vi "Format Library Control VI Info Table.vi"(7 "Methods":T1, 8 "Error in":errorcluster caption="Error in (no error)", 9 "Msg Chain":string, 10 "VI Info Array":T2[](array[typedef]), 11 "VIDoc Printer - Confluence In":refnum<class "VIDoc Printer - Confluence.lvclass">) -> (0 "Error out":errorcluster, 2 "Table String":string, 3 "VIDoc Printer - Confluence Out":refnum<class "VIDoc Printer - Confluence.lvclass">)   [LabVIEW 2023, in "VIDoc Printer - Confluence.lvlib" / "VIDoc Printer - Confluence.lvclass"]
uses:
  VIDoc Printer - Confluence.lvclass
  Parsing/TypeDefs/Method Spec Cluster.ctl
  Parsing/TypeDefs/VI Type Extended Enum.ctl
  <vilib>/picture/picture.llb/imagedata.ctl
  Parsing/TypeDefs/Class Dispatch Type Enum.ctl
  Parsing/TypeDefs/Controls Info Cluster.ctl
  <vilib>/Utility/miscctls.llb/LVKeyTypeDef.ctl
  <vilib>/Utility/miscctls.llb/LVPointTypeDef.ctl
  Parsing/SubVIs/Structure Reporter/Tree Cluster.ctl
  Settings/Printer Settings/Detail Level Enum.ctl
  C:/projects/DMC/Tooling/Git-Action-Service/Source/Documentation Generation/Printers/Printer/VIDoc Printer.lvclass
  VIDoc Printer - Confluence.lvclass/VIDoc Printer - Confluence.ctl
  Printer/VIDoc Printer.lvclass/VIDoc Printer.ctl
  Printer/Accessors/Get Formatting Settings - Bookmark Options.vi
  Accessors/Get Temporary Image Directory+.vi
  Accessors/Get Control Method Column Ordering - Full.vi
  Accessors/Get Control Method Column Ordering - Minimal.vi
  Accessors/Get Control Method Column Ordering - Standard.vi
  Accessors/Get Sortable Tables.vi
  <vilib>/Utility/libraryn.llb/Create Directory Recursive.vi
  Printer/VIDoc Printer.lvclass
  Confluence Formatting/Confluence Formatting.lvlib
  UI Interaction/UI Interaction.lvclass
  C:/projects/DMC/Tooling/Git-Action-Service/Source/Documentation Generation/Printers/Confluence Printer/VIDoc Printer - Confluence.lvclass
  Parsing/VIDoc Parsing.lvlib
  Settings/Printer Settings/Printer Settings.lvclass
  Parsing/SubVIs/Structure Reporter/Structure Reporter.lvlib
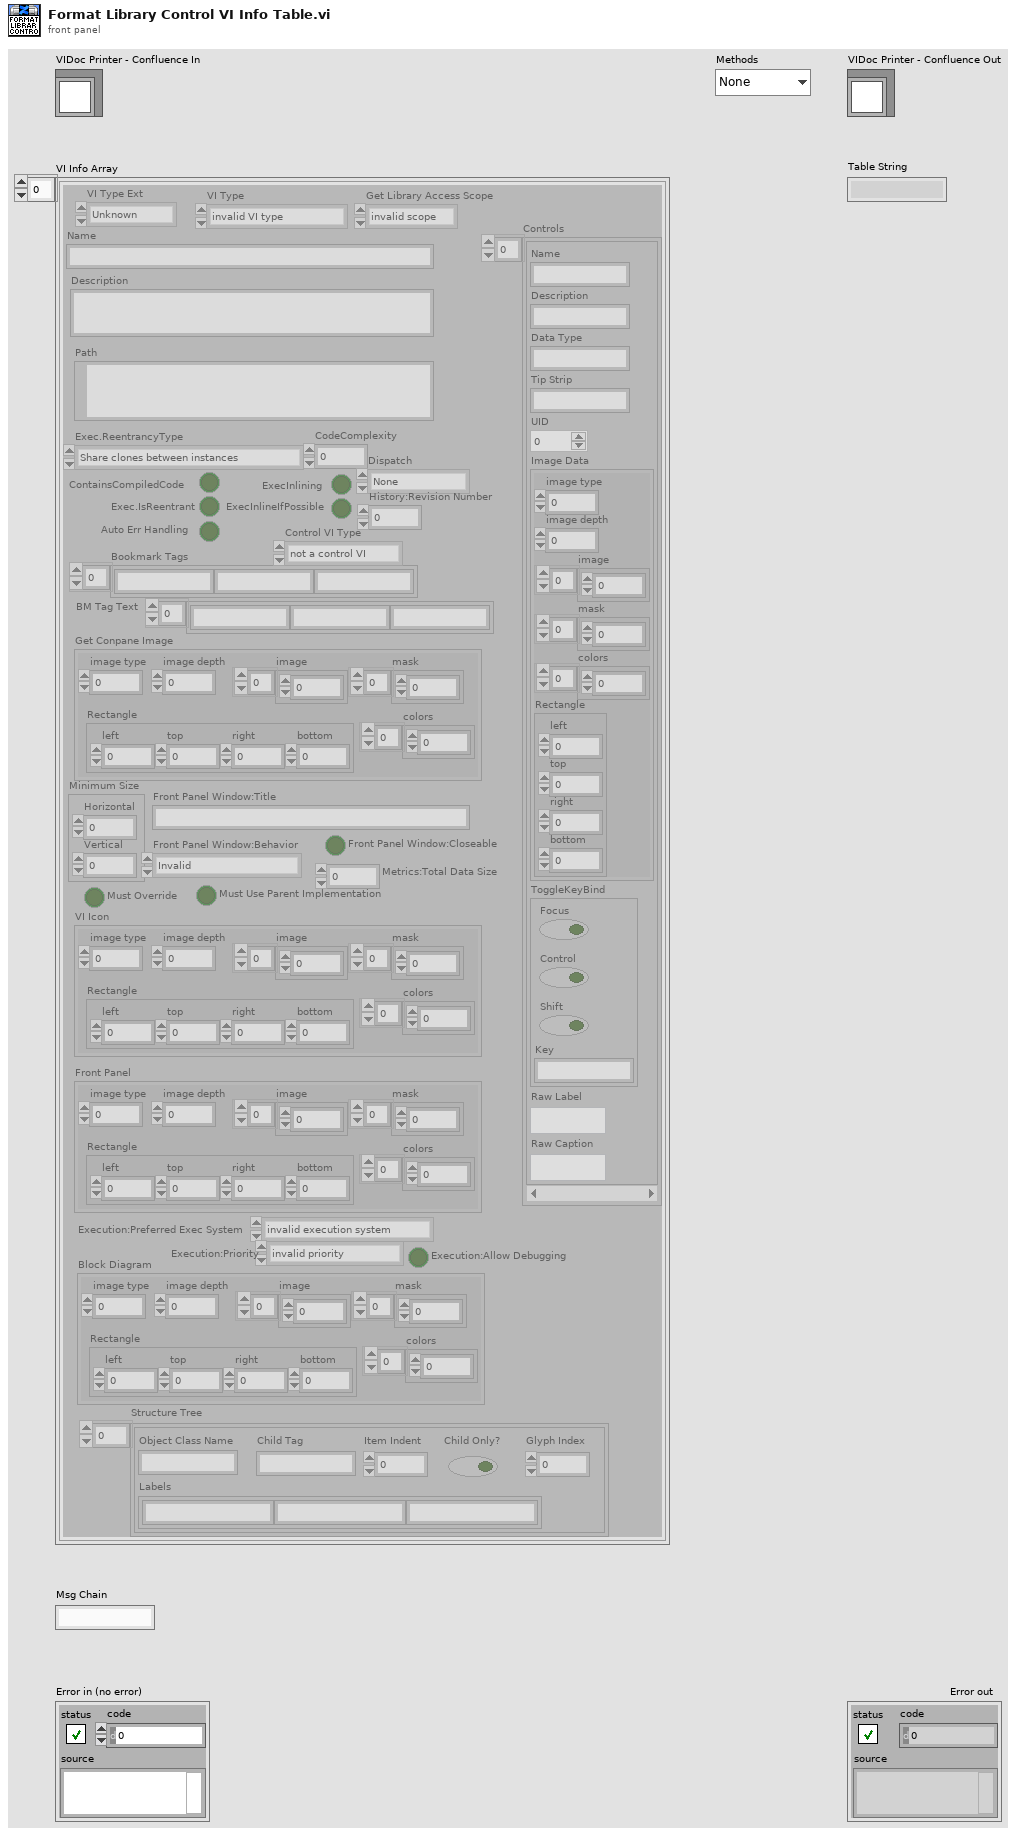
[diagram p1: front panel]
types:
  T1 = typedef "VIDoc Printer.lvlib/Printer Settings.lvclass/Detail Level Enum.ctl" = enum16{"None", "Minimal", "Standard", "Full"}
  T2 = typedef "VIDoc Parsing.lvlib/Method Spec Cluster.ctl" = cluster{"VI Type Ext":T3, "Name":string, "Path":path, "Get Conpane Image":T4, "Description":string, "Get Library Access Scope":enum32{"invalid scope", "public", "private", "protected", "community"}, "Dispatch":T5, "ContainsCompiledCode":bool, "Exec.IsReentrant":bool, "Exec.ReentrancyType":enum16{"Share clones between instances", "Preallocate clone for each instance"}, "ExecInlining":bool, "ExecInlineIfPossible":bool, "Auto Err Handling":bool, "CodeComplexity":sgl, "Bookmark Tags":string[], "Control VI Type":enum32{"not a control VI", "control", "typedef", "strict typedef"}, "Controls":T6[], "VI Type":enum32{"invalid VI type", "Standard VI", "Control VI", "Global VI", "Polymorphic VI", "Configuration VI", "SubSystem", "Facade VI", "Method VI", "Statechart Diagram VI"}, "Minimum Size":T8, "Front Panel Window:Title":string, "Front Panel Window:Behavior":enum32{"Invalid", "Default", "Floating", "Floating/Auto-Hide", "Modal"}, "Front Panel Window:Closeable":bool, "Must Override":bool, "Must Use Parent Implementation":bool, "VI Icon":T4, "Front Panel":T4, "History:Revision Number":u32, "Metrics:Total Data Size":u32, "Execution:Allow Debugging":bool, "Execution:Preferred Exec System":enum32{"invalid execution system", "user interface", "standard", "instrument i/o", "data acquisition", "other 1", "other 2", "same as caller"}, "Execution:Priority":enum32{"invalid priority", "background priority", "normal priority", "above normal priority", "high priority", "time critical priority", "subroutine"}, "BM Tag Text":string[], "Block Diagram":T4, "Structure Tree":T9[]}
  T3 = typedef "VIDoc Parsing.lvlib/VI Type Extended Enum.ctl" = enum16{"Unknown", "Class Method", "Class Accessor Get", "Class Accessor Set", "Class Control", "Library Method", "Library Control", "VI", "Control"}
  T4 = typedef "imagedata.ctl" = cluster{"image type":i32, "image depth":i32, "image":u8[], "mask":u8[], "colors":u32[], "Rectangle":cluster{"left":i16, "top":i16, "right":i16, "bottom":i16}}
  T5 = typedef "VIDoc Parsing.lvlib/Class Dispatch Type Enum.ctl" = enum16{"None", "Static", "Dynamic"}
  T6 = typedef "VIDoc Parsing.lvlib/Controls Info Cluster.ctl" = cluster{"Name":string, "Description":string, "Data Type":string, "Tip Strip":string, "UID":i32, "Image Data":T4, "ToggleKeyBind":T7, "Raw Label":string, "Raw Caption":string}
  T7 = typedef "LVKeyTypeDef.ctl" = cluster{"Focus":bool, "Control":bool, "Shift":bool, "Key":string}
  T8 = typedef "LVPointTypeDef.ctl" = cluster{"Horizontal":i16, "Vertical":i16}
  T9 = typedef "VIDoc Parsing.lvlib/Structure Reporter.lvlib/Tree Cluster.ctl" = cluster{"Object Class Name":string, "Labels":string[], "Child Tag":string, "Item Indent":i32, "Child Only?":bool, "Glyph Index":i32}
  T10 = enum32{"invalid scope", "public", "private", "protected", "community"}
  T11 = enum32{"not a control VI", "control", "typedef", "strict typedef"}
  T12 = typedef "VIDoc Printer.lvlib/Printer Settings.lvclass/Bookmark Options.ctl" = cluster{"Bookmarks as New Line in VI Descriptions":bool, "Unique Bookmark Tags Only":bool, "Include Tag and Text":bool}
  T13 = typedef "VIDoc Printer - Confluence.lvlib/VIDoc Settings - Confluence.lvclass/VI Info Column.ctl" = enum16{"Name", "Conpane", "BD", "FP", "VI Icon", "Description", "Reentrant", "Inline", "Auto Error", "Compiled", "Code Complexity", "Data Size", "Debug", "Priority", "Rev", "Minimum Size", "Title", "FP Behavior", "FP Closeable", "Author", "Commit Hash", "Last Change", "Branch", "Scope", "Type", "Dispatch", "Must Override", "Must Use Parent", "Structure Tree"}
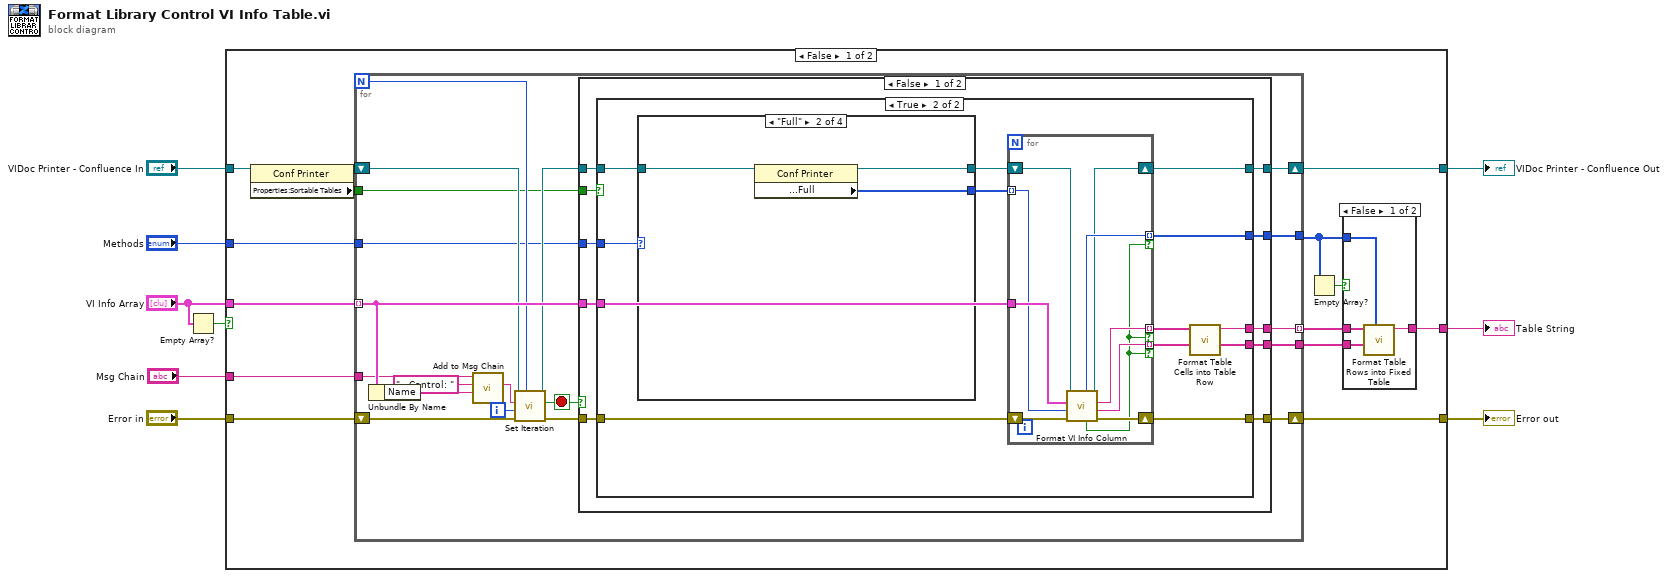
[diagram p0: block diagram]
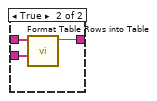
[diagram p2: hidden frame]
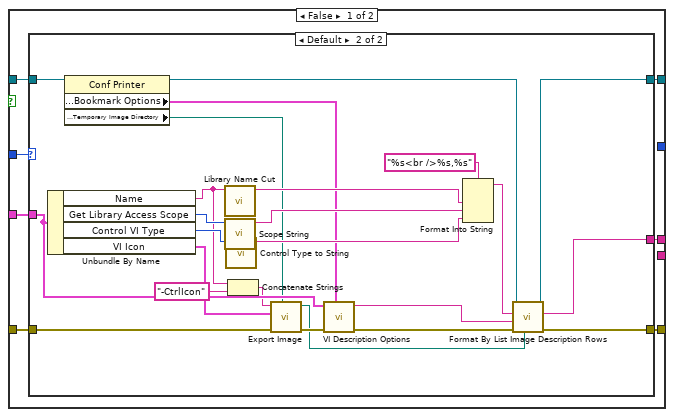
[diagram p3: hidden frame]
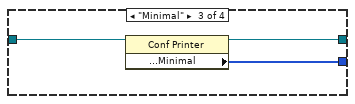
[diagram p6: hidden frame]
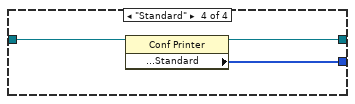
[diagram p7: hidden frame]
diagram:
  n1 = Empty Array?(array="VI Info Array") -> (empty?=w1:bool)
  n2 = case shown="False" w1 {
    tunnel: "Error in" -> [w23 w127]
    tunnel: [w22 w127] -> w8
    tunnel: [w21 _] -> w7
    tunnel: "VI Info Array" -> [w20 _]
    tunnel: "VIDoc Printer - Confluence In" -> [w19 w128]
    tunnel: [w18 w128] -> w5
    tunnel: "Msg Chain" -> [w17 _]
    tunnel: "Methods" -> [w16 _]
    frame False {
      n3 = property class="Conf Printer"(reference=w19) -> (reference out=w11:refnum<class "VIDoc Printer - Confluence.lvclass">, "Properties:Sortable Tables"=w10:bool)  [unwired: 1 in, 1 out]
      n4 = for {
        N -> [w40]
        tunnel: w20 -> [w43] mode=indexing
        shift-right: [w49] -> w18
        shift-left: w11 -> [w38]
        shift-right: [w48] -> w22
        shift-left: w23 -> [w45]
        tunnel: w17 -> [w41]
        tunnel: w16 -> [w35]
        tunnel: [w34] -> w15 mode=indexing
        tunnel: [w33] -> w14
        tunnel: [w32] -> w12
        tunnel: w10 -> [w31]
        i -> [w39]
        stop <- w36 stop-if-true
        n5 = Unbundle By Name(w43) -> ("Name"=w42:string)
        n6 = call "Add to Msg Chain.vi"("New"=w42, "Separator (-)"=" - Control: ", "Msg Chain in"=w41) -> ("Msg Chain out"=w46:string)  [unwired: 8 in]
        n7 = call "Set Iteration.vi"("Progress Max"=w40, "error in (no error)"=w45, "Progress Value"=w39, "Message (No Message Update)"=w46, "VIDoc Printer In"=w38) -> ("error out"=w44:errorcluster, "Abort?"=w36:bool, "VIDoc Printer Out"=w37:refnum<class "VIDoc Printer - Confluence.lvclass">)  [unwired: 4 in]
        n8 = case shown="False" w36 {
          tunnel: [w59 w126] -> w49
          tunnel: [w58 w125] -> w48
          tunnel: w44 -> [w57 w125]
          tunnel: w43 -> [w56 _]
          tunnel: w37 -> [w55 w126]
          tunnel: w35 -> [w54 _]
          tunnel: [w53 _] -> w34
          tunnel: [w52 _] -> w33
          tunnel: [w51 _] -> w32
          tunnel: w31 -> [w50 _]
          frame False {
            n9 = case shown="True" w50 {
              tunnel: [w66 w99] -> w59
              tunnel: [w65 w103] -> w58
              tunnel: w57 -> [w64 w98]
              tunnel: w56 -> [w63 w97]
              tunnel: w55 -> [w62 w93]
              tunnel: w54 -> [w61 w96]
              tunnel: [w60 w102] -> w53
              tunnel: [_ w101] -> w52
              tunnel: [_ w100] -> w51
              frame False {
                n10 = case shown="Default" w61 {
                  tunnel: [w68 w84] -> w66
                  tunnel: [w67 w82] -> w65
                  tunnel: w64 -> [w67 w87]
                  tunnel: w63 -> [_ w92]
                  tunnel: w62 -> [w68 w85]
                  tunnel: [_ w78] -> w60
                  frame "None" {
                  }
                  frame Default {
                    n11 = Unbundle By Name(w92) -> ("Name"=w73:string, "Get Library Access Scope"=w91:T10, "Control VI Type"=w90:T11, "VI Icon"=w80:T4)
                    n12 = property class="Conf Printer"(reference=w85) -> (reference out=w76:refnum<class "VIDoc Printer - Confluence.lvclass">, "Properties:Settings:Formatting Options:Bookmark Options"=w75:T12, "Properties:Temporary Image Directory"=w69:path)  [unwired: 1 in, 1 out]
                    n13 = call "Library Name Cut.vi"("Name in"=w73) -> ("Name out"=w77:string)  [unwired: 10 in]
                    n14 = call "Scope String.vi"("Get Library Access Scope"=w91) -> ("String"=w89:string)  [unwired: 10 in]
                    n15 = call "Control Type to String.vi"("Control VI Type"=w90) -> ("String"=w88:string)  [unwired: 10 in]
                    n16 = Concatenate Strings(w73, "-CtrlIcon" ("string")) -> (w72:string)
                    n17 = call "Export Image.vi"("Temporary Image Directory"=w69, "Error in"=w87, "Image Data"=w80, "Name"=w72) -> ("Error out"=w86:errorcluster, "Image Path"=w79:path)  [unwired: 6 in]
                    n18 = call "VI Description Options.vi"("Bookmark Options"=w75, "Error in"=w86, "VI Info"=w92) -> ("Error out"=w83:errorcluster, "Description"=w81:string)  [unwired: 7 in]
                    n19 = Format Into String(format string="%s<br />%s,%s", w77, w89, w88) -> (resulting string=w70:string)  [unwired: 2 in, 1 out]
                    n20 = call "Format By List Image Description Rows.vi"("Image"=w79, "error in (no error)"=w83, "Description"=w81, "Name"=w70, "VIDoc Printer - Confluence In"=w76) -> ("error out"=w82:errorcluster, "Table Rows Text"=w78:string, "VIDoc Printer - Confluence Out"=w84:refnum<class "VIDoc Printer - Confluence.lvclass">)  [unwired: 3 in, 1 out]
                  }
                }
              }
              frame True {
                n21 = case shown="\"Full\"" w96 {
                  tunnel: [_ w106 w109 w112] -> w95
                  tunnel: [w105 w107 w110 w113] -> w94
                  tunnel: w93 -> [w105 w108 w111 w114]
                  frame "None" {
                  }
                  frame "Full" {
                    n22 = property class="Conf Printer"(reference=w108) -> (reference out=w107:refnum<class "VIDoc Printer - Confluence.lvclass">, "Properties:Table Column Ordering:Control Method:Full"=w106:T13[])  [unwired: 1 in, 1 out]
                  }
                  frame "Minimal" {
                    n23 = property class="Conf Printer"(reference=w111) -> (reference out=w110:refnum<class "VIDoc Printer - Confluence.lvclass">, "Properties:Table Column Ordering:Control Method:Minimal"=w109:T13[])  [unwired: 1 in, 1 out]
                  }
                  frame "Standard" {
                    n24 = property class="Conf Printer"(reference=w114) -> (reference out=w113:refnum<class "VIDoc Printer - Confluence.lvclass">, "Properties:Table Column Ordering:Control Method:Standard"=w112:T13[])  [unwired: 1 in, 1 out]
                  }
                }
                n25 = for {
                  shift-right: [w123] -> w103
                  shift-left: w98 -> [w124]
                  tunnel: [w122] -> w101 mode=indexing if=w115
                  tunnel: [w121] -> w104 mode=indexing if=w115
                  tunnel: [w120] -> w100 mode=indexing if=w115
                  shift-right: [w118] -> w99
                  shift-left: w94 -> [w119]
                  tunnel: w97 -> [w117]
                  tunnel: w95 -> [w116] mode=indexing
                  n26 = call "Format VI Info Column.vi"("error in (no error)"=w124, "Column"=w116, "VI Info"=w117, "VIDoc Printer - Confluence In"=w119) -> ("error out"=w123:errorcluster, "Header"=w122:string, "Cell Text"=w121:string, "VIDoc Printer - Confluence Out"=w118:refnum<class "VIDoc Printer - Confluence.lvclass">, "Viable Value?"=w115:bool, "Pixel Width"=w120:i16)  [unwired: 2 in]
                }
                n27 = call "Format Table Cells into Table Row.vi"("Table Cells"=w104) -> ("Table Row Text"=w102:string)  [unwired: 10 in]
              }
            }
          }
          frame True {
          }
        }
      }
      n28 = Empty Array?(array=w12) -> (empty?=w13:bool)
      n29 = case shown="False" w13 {
        tunnel: [w25 w30] -> w21
        tunnel: w15 -> [w26 w29]
        tunnel: w14 -> [w27 w28]
        tunnel: w12 -> [w24 _]
        frame False {
          n30 = call "Format Table Rows into Fixed Table.vi"("Column Pixel Widths"=w24, "Table Headers"=w27, "Table Rows"=w26) -> ("Table Text"=w25:string)  [unwired: 8 in]
        }
        frame True {
          n31 = call "Format Table Rows into Table.vi"("Table Headers"=w28, "Table Rows"=w29) -> ("Table Text"=w30:string)  [unwired: 9 in]
        }
      }
    }
    frame True {
    }
  }
  "Error out" <- w8
  "Table String" <- w7
  "VIDoc Printer - Confluence Out" <- w5
